vi "Launch Subscriber.vi"(8 "error in (no error)":errorcluster, 10 "Actor to Launch":refnum<class "Actor.lvclass">, 11 "Publisher in":refnum<class "Publisher.lvclass">) -> (0 "error out":errorcluster, 3 "Publisher out":refnum<class "Publisher.lvclass">)   [LabVIEW 2020, in "Publisher.lvlib" / "Publisher.lvclass"]
doc: "Launch a subscribing actor placing registering the actor enqueuer both by ID and by Actor.\n\nAlso obtains an enqueuer named notifier."
uses:
  Publisher.lvclass
  PPL/HDH.Actor Framework.Core.Actor.lvlibp/1abvi3w/vi.lib/ActorFramework/Actor/Actor.lvclass
  Publisher.lvclass/Publisher.ctl
  Add Subscriber.vi/9bfa7042-f496-41a0-bdb3-f05adf9a1a12.vi
  PPL/HDH.Actor Framework.Core.Utility.lvlibp/Object/To Default Object.vi
  PPL/HDH.Actor Framework.Core.Actor.lvlibp/1abvi3w/vi.lib/ActorFramework/Message Enqueuer/Message Enqueuer.lvclass
  PPL/HDH.Data.Generic.lvlibp/Synchronization/Notifier/Notifier.lvclass
  PPL/HDH.Actor Framework.Core.Utility.lvlibp
  C:/Current projects/WS/PPL/HDH.Actor Framework.Core.Actor.lvlibp/1abvi3w/vi.lib/ActorFramework/Actor/Actor.lvclass
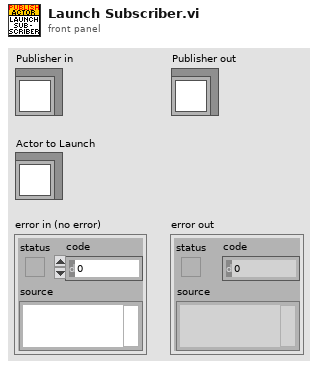
[diagram p1: front panel]
types:
  T1 = typedef "Publisher.lvlib/Publisher.lvclass/Ctl_Subscription Element.ctl" = cluster{"Object":refnum<class>, "Enqueuers":refnum<class "Message Enqueuer.lvclass">[]}
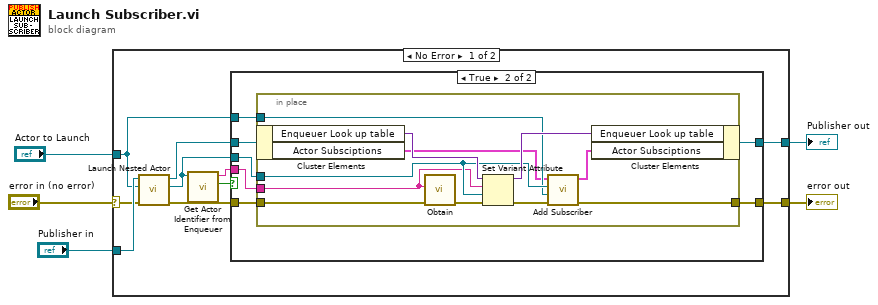
[diagram p0: block diagram]
diagram:
  n1 = case shown="No Error" "error in (no error)" {
    selector: "error in (no error)" -> [w7 w37]
    tunnel: [w9 w37] -> w4
    tunnel: [w10 w36] -> w2
    tunnel: "Publisher in" -> [w15 w36]
    tunnel: "Actor to Launch" -> [w8 _]
    frame No Error {
      n2 = call "Launch Nested Actor.vi"("error in (no error)"=w7, "Nested Actor"=w8, "Caller Actor in"=w15) -> ("error out"=w11:errorcluster, "Nested Actor's Enqueuer"=w12:refnum<class "Message Enqueuer.lvclass">, "Caller Actor out"=w14:refnum<class "Publisher.lvclass">)  [unwired: 6 in]
      n3 = call "Get Actor Identifier from Enqueuer.vi"("Message Enqueuer in"=w12) -> ("Valid Enqueuer?"=w6:bool, "Actor ID string out"=w13:string)  [unwired: 9 in]
      n4 = case shown="True" w6 {
        tunnel: w14 -> [w17 w24]
        tunnel: w13 -> [_ w23]
        tunnel: w12 -> [_ w22]
        tunnel: w11 -> [w16 w21]
        tunnel: [w17 w20] -> w10
        tunnel: [w16 w19] -> w9
        tunnel: w8 -> [_ w18]
        frame False {
        }
        frame True {
          n5 = in-place {
            in-place-border: w23 -> [w27]
            in-place-border: w22 -> [w32]
            in-place-border: w21 -> [w26]
            in-place-border: [w30] -> w19
            in-place-border: w18 -> [w29]
            n6 = in-place-cluster #1(w24) -> ("Enqueuer Look up table"=w35:variant, "Actor Subsciptions"=w28:T1[])
            n7 = call "Obtain.vi"("error in (no error)"=w26, "Name (\"\")"=w27) -> ("error out"=w25:errorcluster)  [unwired: 7 in, 2 out]
            n8 = Set Variant Attribute(Variant=w35, name=w27, value=w32, error in=w25) -> (Variant out=w34:variant, error out=w31:errorcluster)  [unwired: 1 out]
            n9 = call "Add Subscriber.vi"("error in (no error)"=w31, "Subscription Object"=w29, "Subscriber Enqueuer"=w32, "Subsciptions in"=w28) -> ("error out"=w30:errorcluster, "Subsciptions out"=w33:T1[])  [unwired: 6 in]
            n10 = in-place-cluster #1("Enqueuer Look up table"=w34, "Actor Subsciptions"=w33) -> (w20:refnum<class "Publisher.lvclass">)
          }
        }
      }
    }
    frame Error {
    }
  }
  "error out" <- w4
  "Publisher out" <- w2
